vi "Get Class KeyValueType.vi"(8 "error in (no error)":errorcluster, 10 "class":refnum<class "_ISerializable.lvclass">, 11 "ORM Scripter in":refnum<class "ORM Scripter.lvclass">) -> (0 "error out":errorcluster, 3 "ORM Scripter out":refnum<class "ORM Scripter.lvclass">)   [LabVIEW 2018, in "ORM Scripter.lvclass"]
uses:
  ORM Scripter.lvclass
  _Serializable Base Object/_ISerializable.lvclass
  Typedefs/tablename-cols-type-cluster.ctl
  ORM Scripter.lvclass/ORM Scripter.ctl
  <vilib>/NI/Configuration Framework/class discovery singleton/class discovery singleton.lvlib
  Serializer/Serializer.lvclass
panel:
  out "Array 2":u32[](array[numeric])
  out "Array":string[](array[string])
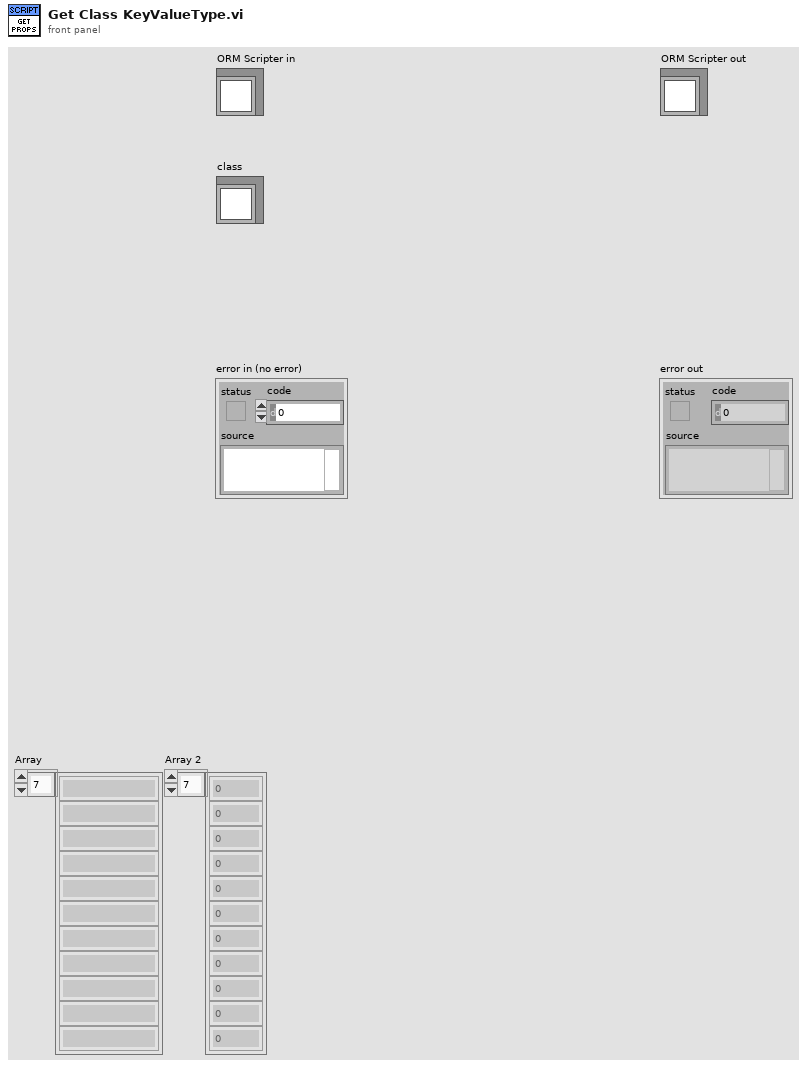
[diagram p1: front panel]
types:
  T1 = typedef "tablename-cols-type-cluster.ctl" = cluster{"table name":string, "col names":string[], "lv type  & representation":string[]}
  T2 = typedef "LVNumericRepresentation.ctl" = enum32{"Extended Precision", "Double Precision", "Single Precision", "Long", "Word", "Byte", "Unsigned Long", "Unsigned Word", "Unsigned Byte", "Complex Extended", "Complex Double", "Complex Single", "Quad", "Unsigned Quad", "Fixed-Point"}
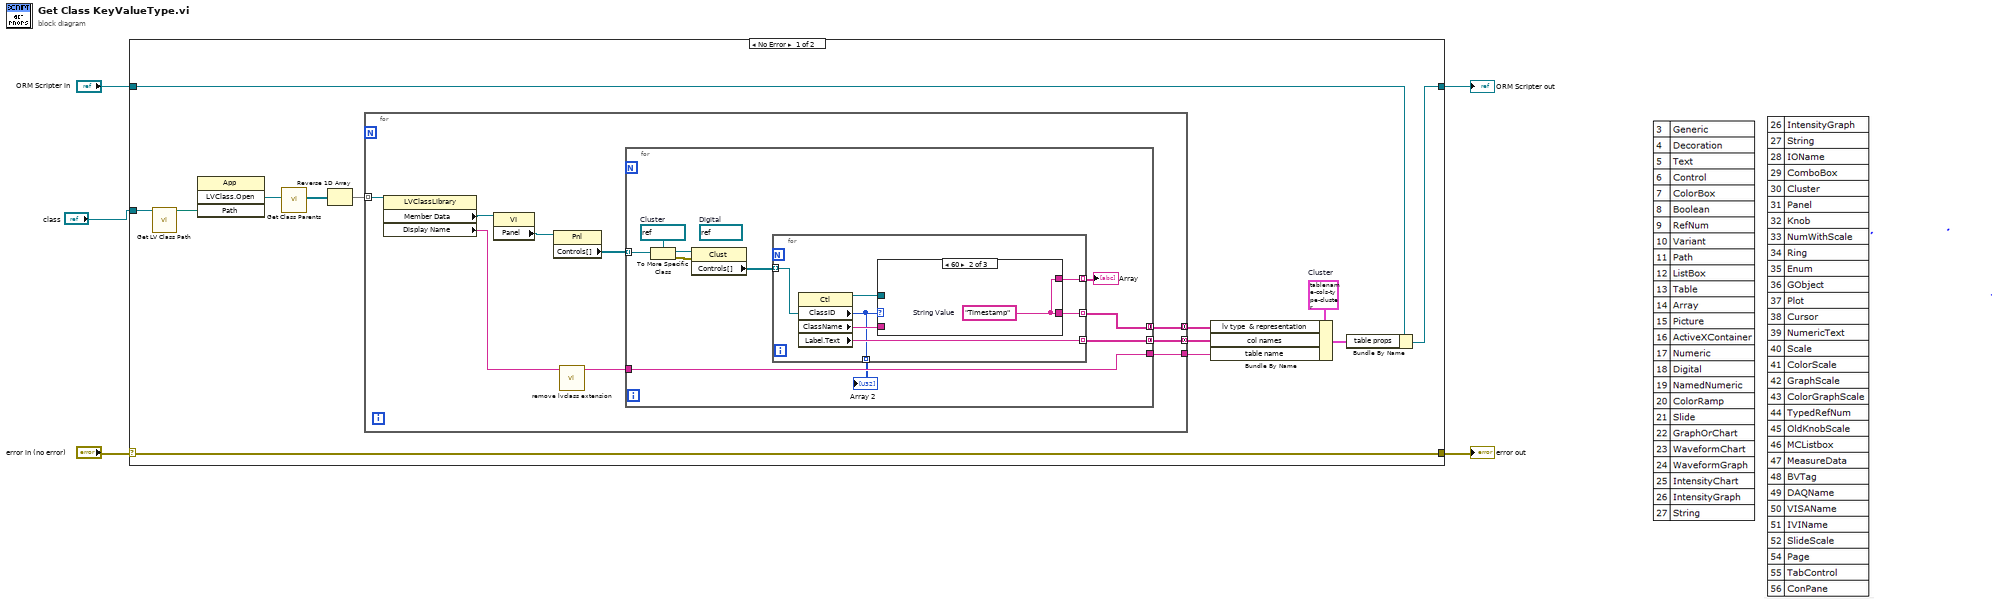
[diagram p0: block diagram]
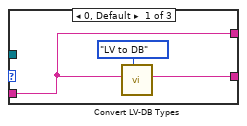
[diagram p2: hidden frame]
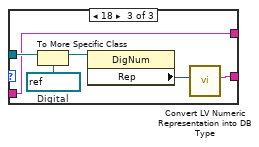
[diagram p3: hidden frame]
diagram:
  n1 = case shown="No Error" "error in (no error)" {
    selector: "error in (no error)" -> [w18 w56]
    tunnel: [w18 w56] -> w4
    tunnel: [w7 w55] -> w2
    tunnel: "ORM Scripter in" -> [w6 w55]
    tunnel: "class" -> [w14 _]
    frame No Error {
      w9 = T1 {"table name"="Product-B.lvclass", "col names"=["uid", "isObsolete", "status"], "lv type  & representation"=["Unsigned Quad", "Boolean", "Unsigned Byte"]}  # Cluster
      n2 = call <vilib>:"Get LV Class Path.vi"("object"=w14) -> ("class path"=w15:path)  [unwired: 9 in, 1 out]
      n3 = invoke class="App" method="LVClass.Open"("Path"=w15) -> ("LVClass.Open"=w17:refnum<vi>)  [unwired: 3 in, 3 out]
      n4 = call "Get Class Parents.vi"("LVClassLibrary in"=w17) -> ("Array"=w16:refnum<vi>[])  [unwired: 9 in, 1 out]
      n5 = Reverse 1D Array(array=w16) -> (reversed array=w13:refnum<vi>[])
      n6 = for {
        tunnel: w13 -> [w24] mode=indexing
        tunnel: [w23] -> w12 mode=concatenating
        tunnel: [w22] -> w11 mode=concatenating
        tunnel: [w21] -> w10
        n7 = property class="LVClassLibrary"(reference=w24) -> ("Member Data"=w26:refnum<vi>, "Display Name"=w20:string)  [unwired: 1 in, 2 out]
        n8 = property class="VI"(reference=w26) -> ("Panel"=w27:refnum<vi>)  [unwired: 1 in, 2 out]
        n9 = property class="Pnl"(reference=w27) -> ("Controls[]"=w25:refnum<vi>[])  [unwired: 1 in, 2 out]
        n10 = call "remove lvclass extension.vi"("class name in"=w20) -> ("class name out"=w19:string)  [unwired: 10 in]
        n11 = for {
          tunnel: w25 -> [w33] mode=indexing
          tunnel: w19 -> [w30]
          tunnel: [w32] -> w23 mode=concatenating
          tunnel: [w31] -> w22 mode=concatenating
          tunnel: [w30] -> w21
          (unwired) refnum<vi> refnum  # Digital
          w37 = refnum<vi> refnum  # Cluster
          n12 = To More Specific Class(target class=w37, reference=w33) -> (specific class reference=w36:refnum<vi>, error out=w35:errorcluster)  [unwired: 1 in]
          n13 = property class="Clust"(reference=w36, error in=w35) -> ("Controls[]"=w34:refnum<vi>[])  [unwired: 2 out]
          n14 = for {
            tunnel: w34 -> [w44] mode=indexing
            tunnel: [w40] -> w31 mode=indexing
            tunnel: [w41] -> w32 mode=indexing
            tunnel: [w39] -> w29 mode=indexing
            tunnel: [w38] -> w28 mode=indexing
            n15 = property class="Ctl"(reference=w44) -> (reference out=w43:refnum<vi>, "ClassID"=w38:u32, "ClassName"=w42:string, "Label.Text"=w40:string)  [unwired: 1 in, 1 out]
            n16 = case shown="60" w38 {
              tunnel: w43 -> [_ _ w52]
              tunnel: w42 -> [w45 _ w49]
              tunnel: [w47 w48 w50] -> w41
              tunnel: [w45 w48 w49] -> w39
              frame 0, Default {
                n17 = call "Convert LV-DB Types.vi"("conversion"=enum16{"LV to DB", "DB to LV"}."LV to DB", "DataType"=w45) -> ("Converted Type"=w47:string)  [unwired: 8 in, 1 out]
              }
              frame 60 {
                w48 = "Timestamp"  # String Value
              }
              frame 18 {
                w54 = refnum<vi> refnum  # Digital
                n18 = To More Specific Class(target class=w54, reference=w52) -> (specific class reference=w53:refnum<vi>)  [unwired: 1 in, 1 out]
                n19 = property class="DigNum"(reference=w53) -> ("Rep"=w51:T2)  [unwired: 1 in, 2 out]
                n20 = call "Convert LV Numeric Representation into DB Type.vi"("Representation"=w51) -> ("String Value"=w50:string)  [unwired: 10 in]
              }
            }
          }
          "Array" <- w29
          "Array 2" <- w28
        }
      }
      n21 = Bundle By Name(cluster=w9, "lv type  & representation"=w12, "col names"=w11, "table name"=w10) -> (w8:T1)
      n22 = Bundle By Name(cluster=w6, "table props"=w8) -> (w7:refnum<class "ORM Scripter.lvclass">)
    }
    frame Error {
    }
  }
  "error out" <- w4
  "ORM Scripter out" <- w2
